vi "NanotecSMCPDDriver.reset.vi"(0 "VISA resource name":refnum<visa-resource-name>, 1 "contollerID":i32=-1, 5 "error in (no error)":errorcluster) -> (14 "VISA resource name out":refnum<visa-resource-name>, 15 "contollerID out":i32=-1, 19 "error out":errorcluster)   [LabVIEW 2014, in "NanotecSMCPDDriver.lvlib"]
doc: "Resets the instrument and then sends a set of default setup commands to the instrument."
uses:
  NanotecSMCPDDriver.lvlib
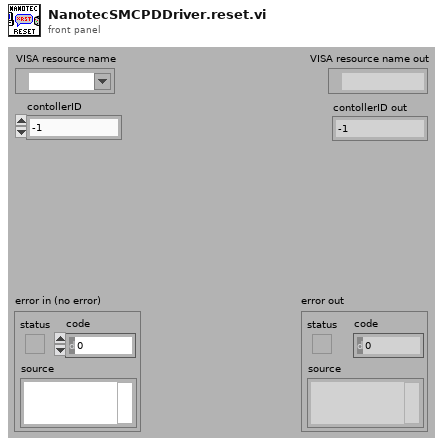
[diagram p1: front panel]
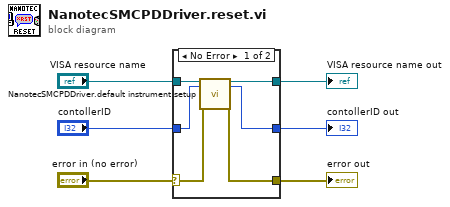
[diagram p0: block diagram]
diagram:
  n1 = case shown="No Error" "error in (no error)" {
    selector: "error in (no error)" -> [w7 w13]
    tunnel: "VISA resource name" -> [w12 w15]
    tunnel: [w11 w15] -> w5
    tunnel: "contollerID" -> [w10 w14]
    tunnel: [w9 w14] -> w3
    tunnel: [w8 w13] -> w2
    frame No Error {
      n2 = call "NanotecSMCPDDriver.default instrument setup.vi"("VISA resource name"=w12, "contollerID"=w10, "error in (no error)"=w7) -> ("VISA resource name out"=w11:refnum<visa-resource-name>, "contollerID out"=w9:i32, "error out"=w8:errorcluster)  [unwired: 14 in]
    }
    frame Error {
    }
  }
  "error out" <- w2
  "VISA resource name out" <- w5
  "contollerID out" <- w3
